vi "ObtainManualModeQueue.vi"(8 "error in (no error)":errorcluster) -> (0 "error out":errorcluster, 3 "queue out":refnum<queue>)   [LabVIEW 2019, in "ManualMode.lvlib"]
uses:
  ManualMode.lvlib
  Cluster - ManualModeMessageCluster.ctl
  Enum - ManualModeMessage.ctl
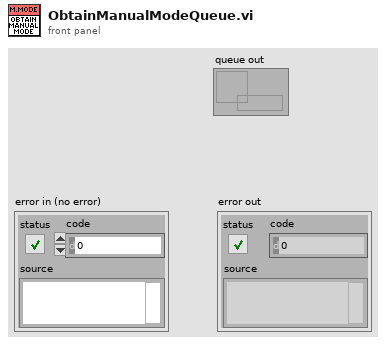
[diagram p1: front panel]
types:
  T1 = typedef "ManualMode.lvlib/Cluster - ManualModeMessageCluster.ctl" = cluster{"Message":T2, "Data":variant}
  T2 = typedef "ManualMode.lvlib/Enum - ManualModeMessage.ctl" = enum16{"Initialize", "Idle", "Start", "Stop", "Pause", "Resume", "BroadcastPreCollection", "MoveCCW", "MoveCW", "StopMove", "SetZero", "GotoZero", "UpdateHW", "Error", "Exit"}
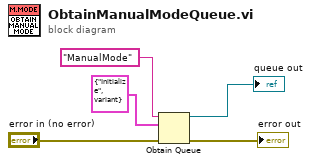
[diagram p0: block diagram]
diagram:
  n1 = Obtain Queue(name (unnamed)="ManualMode", element data type=T1 {"Message"=enum."Initialize", "Data"=variant} ("MessageCluster"), error in (no error)="error in (no error)") -> (queue out=→"queue out":refnum<queue>, error out=→"error out":errorcluster)  [unwired: 2 in, 1 out]
